vi "运维调试_养殖渭水采配水.vi"() -> ()   [LabVIEW 2016, in "PLC.lvlib"]
uses:
  PLC.lvlib
  control/switch.ctl
  <vilib>/Plasmionique/MB Master/MB_Master/MB_Master.lvclass
  <vilib>/Utility/miscctls.llb/LVPointTypeDef.ctl
  <vilib>/Plasmionique/MB Master/MB_Master_Serial/MB_Master_Serial.lvclass
  E:/Program Files (x86)/National Instruments/LabVIEW 2016/vi.lib/Plasmionique/MB Master/MB_Master/MB_Master.lvclass
  <vilib>/Plasmionique/MB Master/MB_Master_TCP/MB_Master_TCP.lvclass
  <vilib>/Plasmionique/MB Master/MB Master.lvlib
panel:
  out "告警":u16(ring) items=["无告警", "液位2异常告警", "进样失败告警", "阀1打开失败告警", "阀1关闭失败告警", "阀2打开失败告警", "阀2关闭失败告警"]
  in  "连接设置":bool
  out "水箱进样超时时间":i16
  out "水箱排液时间":i16
  out "水箱润洗超时时间":i16
  out "Registers":u16[](array[numeric])
  out "状态":u16(ring) items=["空闲", "忙碌"]
  in  "两通阀2":T1
  in  "两通阀1":T1
  out "采配水版本号":string
  out "配水时间":i16
  out "沉淀时间":i16 caption="多参测试、沉淀时间"
  out "管路润洗时间":i16
  out "多列列表框":i32(listbox)
  in  "隔膜泵":T1
  in  "返回":T1
  in  "参数设置":T1
  in  "启动":T1
  in  "停止":T1
  # "S"
  # "S"
  # "S"
  # "S"
  # "S"
  # "S"
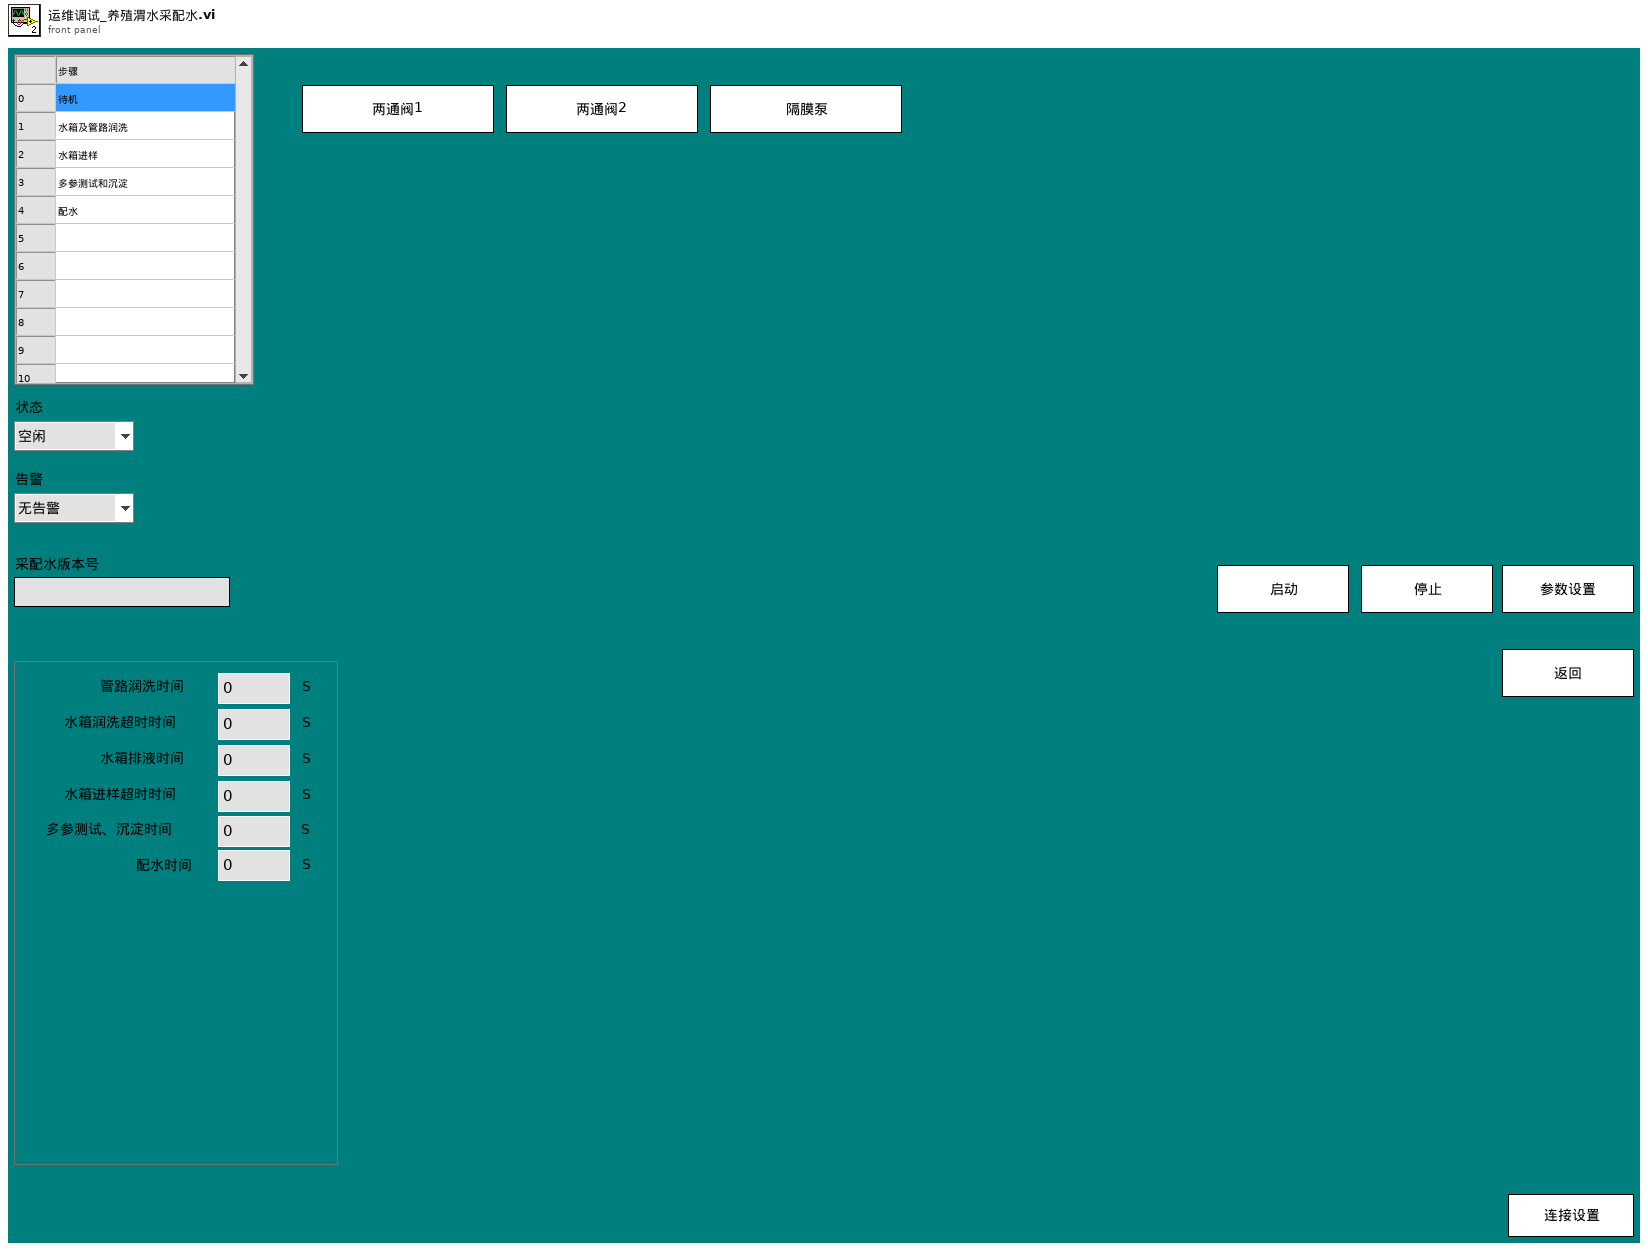
[diagram p1: front panel]
types:
  T1 = typedef "PLC.lvlib/switch.ctl" = bool
  T2 = typedef "参数.ctl" = cluster{"测试模式":enum16{"水样测试", "平行样测试", "集成干预测试", "加标回收"}, "参数启用":T3}
  T3 = typedef "启动参数.ctl" = cluster{"氨氮":bool, "总磷":bool, "总氮":bool, "多参数":bool, "CODmn":bool, "CODCr":bool, "氟化物":bool, "超标留样":bool, "重金属":bool, "挥发酚":bool}
  T4 = typedef "LVPointTypeDef.ctl" = cluster{"Horizontal":i16, "Vertical":i16}
  T5 = cluster{"R0":i16, "R1":i16, "R2":i16, "R3":i16, "R4":i16, "R5":i16, "R6":i16, "R7":i16, "R8":i16, "R9":i16, "R10":i16, "R11":i16, "R12":i16, "R13":i16, "R14":i16, "R15":i16, "R16":i16, "R17":i16, "R18":i16, "R19":i16, "R20":i16, "R21":i16, "R22":i16, "R23":i16, "R24":i16, "R25":i16, "R26":i16, "R27":i16, "R28":i16, "R29":i16, "R30":i16, "R31":i16, "R32":i16, "R33":i16, "R34":i16, "R35":i16, "R36":i16, "R37":i16, "R38":i16, "R39":i16, "R40":i16, "R41":i16, "R42":i16, "R43":i16, "R44":i16, "R45":i16, "R46":i16, "R47":i16, "R48":i16, "R49":i16, "R50":i16, "R51":i16, "R52":i16, "R53":i16, "R54":i16, "R55":i16, "R56":i16, "R57":i16, "R58":i16, "R59":i16, "R60":i16, "R61":i16, "R62":i16, "R63":i16, "R64":i16, "R65":i16, "R66":i16, "R67":i16, "R68":i16, "R69":i16, "R70":i16, "R71":i16, "R72":i16, "R73":i16, "R74":i16, "R75":i16, "R76":i16, "R77":i16, "R78":i16, "R79":i16}
  T6 = cluster{"seconds since 1Jan1904":timestamp, "table输入":string, string, "table输入":string}
  T7 = cluster{"命令":string, cluster{"starting address":u16, "holding register value":u16}}
  T8 = cluster{"命令":string, "数据":cluster{"starting address":u16, "holding register values":u16[]}}
  T9 = cluster{"测试模式":enum16{"水样测试", "平行样测试", "集成干预测试", "加标回收"}, "参数启用":T3}
  T10 = cluster{"baud rate (bps)":u32, "stop bits":u16, "parity":u16, "flow control":u16, "timeout":u32, "retries":i32}
  T11 = cluster{"starting address":u16, "holding register values":u16[]}
  T12 = cluster{"starting address":u16, "holding register value":u16}
  T13 = cluster{"starting address":u16, "coil values":bool[]}
  T14 = cluster{"连接类型":enum16{"串口", "TCP"}, "串口":string, "IP":string, "PORT":u16}
  T15 = cluster{"WORD[0]":u16, "WORD[1]":u16, "WORD[2]":u16, "WORD[3]":u16, "WORD[4]":u16, "WORD[5]":u16, "WORD[6]":u16, "WORD[7]":u16, "WORD[8]":u16, "WORD[9]":u16, "WORD[10]":u16, "WORD[11]":u16, "WORD[12]":u16, "WORD[13]":u16, "WORD[14]":u16, "WORD[15]":u16, "WORD[16]":u16, "WORD[17]":u16, "WORD[18]":u16, "WORD[19]":u16, "WORD[20]":u16, "WORD[21]":u16, "WORD[22]":u16, "WORD[23]":u16, "WORD[24]":u16, "WORD[25]":u16, "WORD[26]":u16, "WORD[27]":u16, "WORD[28]":u16, "WORD[29]":u16, "WORD[30]":u16, "WORD[31]":u16, "WORD[32]":u16, "WORD[33]":u16, "WORD[34]":u16, "WORD[35]":u16, "WORD[36]":u16, "WORD[37]":u16, "WORD[38]":u16, "WORD[39]":u16, "WORD[40]":u16, "WORD[41]":u16, "WORD[42]":u16, "WORD[43]":u16, "WORD[44]":u16, "WORD[45]":u16, "WORD[46]":u16, "WORD[47]":u16, "WORD[48]":u16, "WORD[49]":u16, "WORD[50]":u16, "WORD[51]":u16, "WORD[52]":u16, "WORD[53]":u16, "WORD[54]":u16, "WORD[55]":u16, "WORD[56]":u16, "WORD[57]":u16, "WORD[58]":u16, "WORD[59]":u16, "WORD[60]":u16, "WORD[61]":u16, "WORD[62]":u16, "WORD[63]":u16, "WORD[64]":u16, "WORD[65]":u16, "WORD[66]":u16, "WORD[67]":u16, "WORD[68]":u16, "WORD[69]":u16, "WORD[70]":u16, "WORD[71]":u16, "WORD[72]":u16, "WORD[73]":u16, "WORD[74]":u16, "WORD[75]":u16, "WORD[76]":u16, "WORD[77]":u16, "WORD[78]":u16, "WORD[79]":u16}
  T16 = cluster{"Registers[0]":u16, "Registers[1]":u16, "Registers[2]":u16, "Registers[3]":u16, "Registers[4]":u16, "Registers[5]":u16, "Registers[6]":u16, "Registers[7]":u16, "Registers[8]":u16, "Registers[9]":u16, "Registers[10]":u16, "Registers[11]":u16, "Registers[12]":u16, "Registers[13]":u16, "Registers[14]":u16, "Registers[15]":u16, "Registers[16]":u16, "Registers[17]":u16, "Registers[18]":u16, "Registers[19]":u16, "Registers[20]":u16, "Registers[21]":u16, "Registers[22]":u16, "Registers[23]":u16, "Registers[24]":u16, "Registers[25]":u16, "Registers[26]":u16, "Registers[27]":u16, "Registers[28]":u16, "Registers[29]":u16, "Registers[30]":u16, "Registers[31]":u16, "Registers[32]":u16, "Registers[33]":u16, "Registers[34]":u16, "Registers[35]":u16, "Registers[36]":u16}
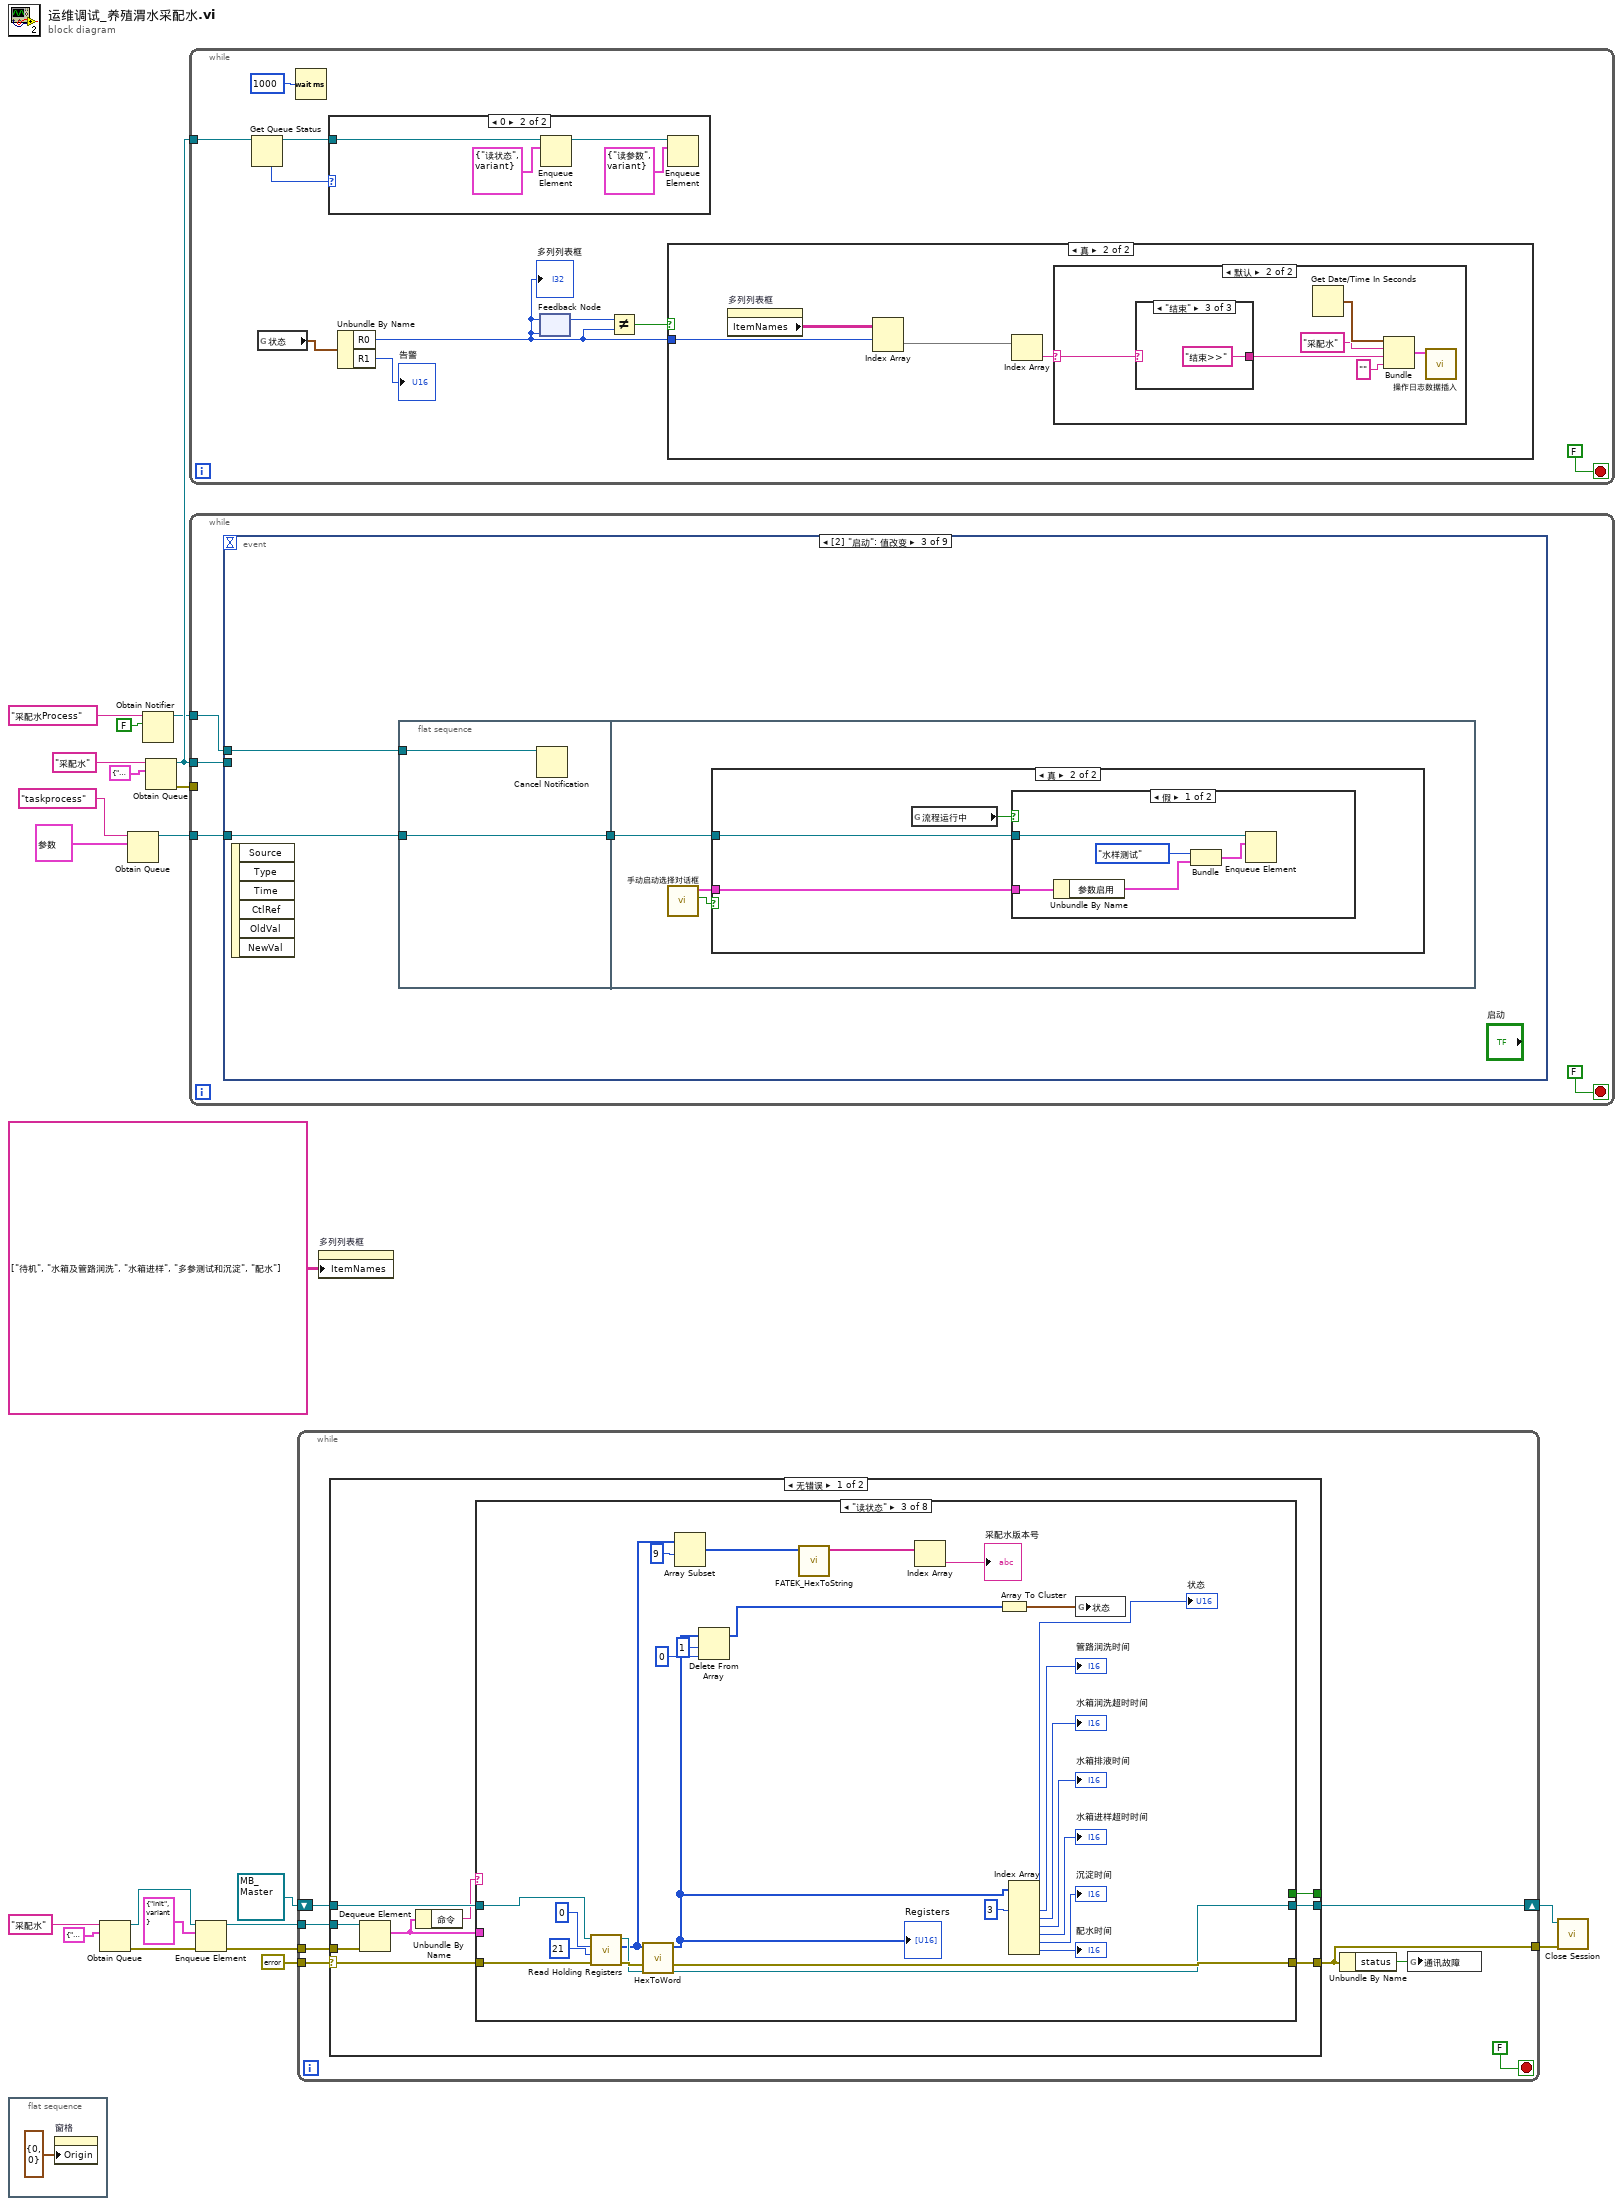
[diagram p0: block diagram]
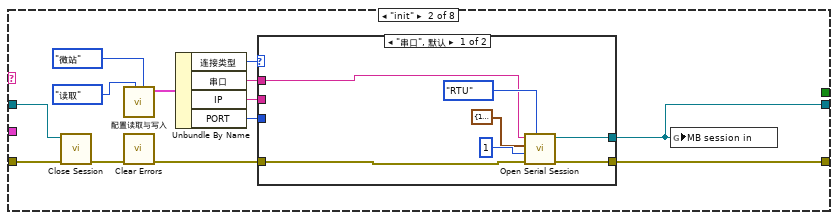
[diagram p3: hidden frame]
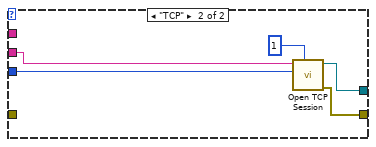
[diagram p4: hidden frame]
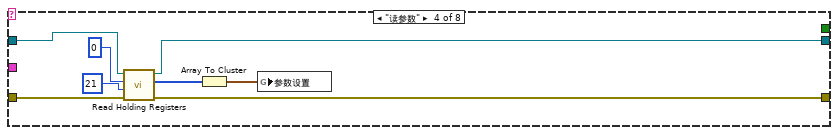
[diagram p5: hidden frame]
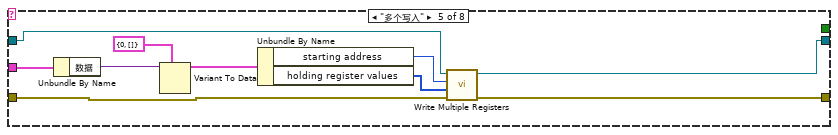
[diagram p6: hidden frame]
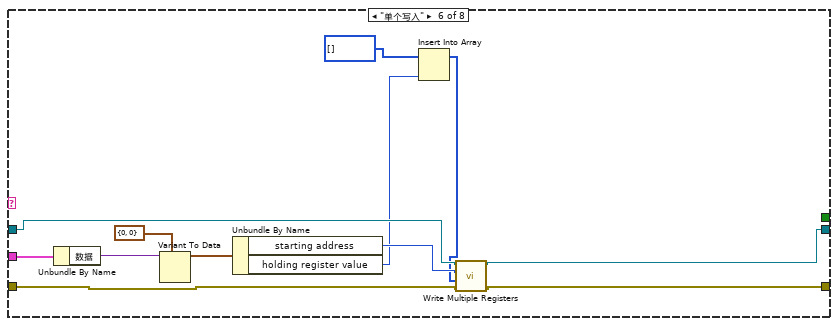
[diagram p7: hidden frame]
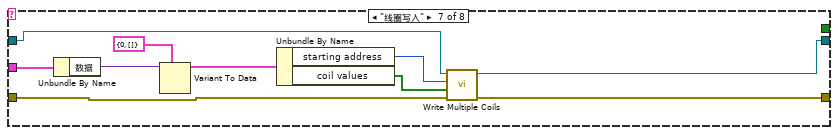
[diagram p8: hidden frame]
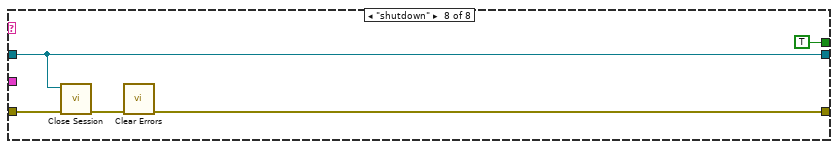
[diagram p9: hidden frame]
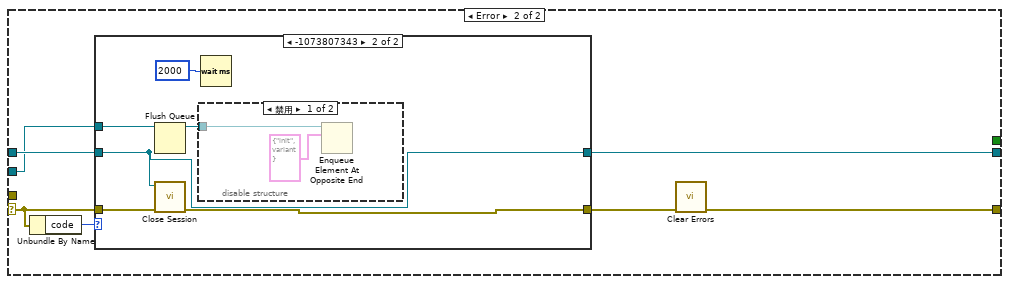
[diagram p10: hidden frame]
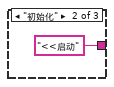
[diagram p17: hidden frame]
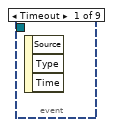
[diagram p18: hidden frame]
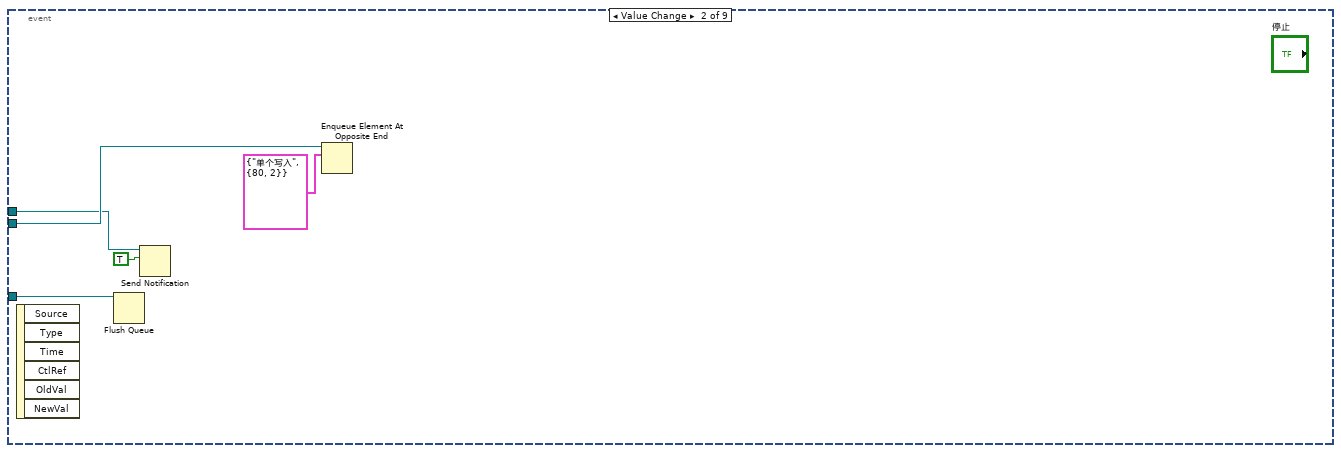
[diagram p19: hidden frame]
diagram:
  n1 = flat-sequence {
    frame #0 {
      n2 = property on="窗格" class="Pane"("Origin"=T4 {"Horizontal"=0, "Vertical"=0} ("原点")) -> ()  [unwired: 2 in, 2 out]
    }
  }
  n3 = Obtain Queue(name (unnamed)="采配水" ("名称（未命名）"), element data type=cluster{"命令":string, "数据":variant} {"命令"="", "数据"=variant}) -> (queue out=w12:refnum<queue>, error out=w11:errorcluster)  [unwired: 3 in, 1 out]
  n4 = Obtain Queue(name (unnamed)="taskprocess" ("名称（未命名）"), element data type=T2 {"测试模式"=enum."水样测试", "参数启用"={"氨氮"=FALSE, "总磷"=FALSE, "总氮"=FALSE, "多参数"=FALSE, "CODmn"=FALSE, "CODCr"=FALSE, "氟化物"=FALSE, "超标留样"=FALSE, "重金属"=FALSE, "挥发酚"=FALSE}} ("参数")) -> (queue out=w2:refnum<queue>)  [unwired: 3 in, 2 out]
  n5 = Obtain Notifier(name (unnamed)="采配水Process" ("名称（未命名）"), notification data type=FALSE) -> (notifier out=w15:refnum<notifier>)  [unwired: 2 in, 2 out]
  n6 = Obtain Queue(name (unnamed)="采配水" ("名称（未命名）"), element data type=cluster{"命令":string, "数据":variant} {"命令"="", "数据"=variant}) -> (queue out=w19:refnum<queue>, error out=w20:errorcluster)  [unwired: 3 in, 1 out]
  n7 = while {
    tunnel: w19 -> [w32]
    stop <- FALSE stop-if-true
    n8 = Get Queue Status(queue=w32) -> (queue out=w27:refnum<queue>, # elements in queue=w26:i32)  [unwired: 2 in, 6 out]
    n9 = global read "采配水全局变量.vi" "状态"() -> (w31:T5)
    n10 = Wait (ms)(milliseconds to wait=u32 1000 ("等待时间（毫秒）")) -> ()  [unwired: 1 out]
    n11 = case shown="0" w26 {
      tunnel: w27 -> [_ w37]
      frame Default {
      }
      frame 0 {
        n12 = Enqueue Element(queue=w37, element=cluster{"命令":string, "数据":variant} {"命令"="读状态", "数据"=variant} ("元素")) -> (queue out=w34:refnum<queue>)  [unwired: 2 in, 2 out]
        n13 = Enqueue Element(queue=w34, element=cluster{"命令":string, "数据":variant} {"命令"="读参数", "数据"=variant} ("元素")) -> ()  [unwired: 2 in, 3 out]
      }
    }
    n14 = Unbundle By Name(w31) -> ("R0"=w25:i16, "R1"=→"告警":i16)
    "多列列表框" <- w25
    n15 = feedback-in #1(w25) -> ()
    n16 = feedback #1(w25) -> (w28:i16)
    n17 = Not Equal?(x=w28, y=w25) -> (x != y?=w30:bool)
    n18 = case shown="真" w30 {
      tunnel: w25 -> [_ w40]
      frame False {
      }
      frame True {
        n19 = property on="多列列表框" class="MCListbox (严格)"() -> ("ItemNames"=w41:string[][])  [unwired: 2 in, 2 out]
        n20 = Index Array(array=w41, index (row)=w40) -> (element=w39:string[])  [unwired: 1 in]
        n21 = Index Array(array=w39) -> (element=w38:string)  [unwired: 1 in]
        n22 = case shown="默认" w38 {
          selector: w38 -> [_ w44]
          frame "待机" {
          }
          frame Default {
            n23 = case shown="\"结束\"" w44 {
              selector: w44 -> [w48 _ _]
              tunnel: [w48 "<<启动" "结束>>"] -> w43
              frame Default {
              }
              frame "初始化" {
              }
              frame "结束" {
              }
            }
            n24 = Get Date/Time In Seconds() -> (seconds since 1Jan1904=w47:timestamp)
            n25 = Bundle("seconds since 1Jan1904"=w47, "table输入"="采配水", w43, "table输入"="") -> (w42:T6)  [unwired: 1 in]
            n26 = call "操作日志数据插入.vi"("data"=w42) -> ()  [unwired: 9 in, 1 out]
          }
        }
      }
    }
  }
  n27 = while {
    tunnel: w19 -> [w53]
    tunnel: w20 -> [_]
    tunnel: w15 -> [w52]
    tunnel: w2 -> [w51]
    stop <- FALSE stop-if-true
    n28 = event shown="[2] \"启动\": 值改变" {
      selector: _ -> [_ _ _ _ _ _ _ _ _]
      dyn-events: _ -> [_ _ _ _ _ _ _ _ _]
      timeout: _ -> [_ _ _ _ _ _ _ _ _]
      tunnel: w53 -> [_ w58 _ w85 w98 _ _ _ w110]
      tunnel: w52 -> [_ w57 w62 _ _ _ _ _ _]
      tunnel: w51 -> [_ w55 w60 _ _ _ _ _ _]
      event Timeout {
        n29 = event-data() -> ()  [unwired: 1 in, 3 out]
      }
      event Value Change {
        n30 = event-data() -> ()  [unwired: 1 in, 6 out]
        n31 = Flush Queue(queue=w55) -> ()  [unwired: 1 in, 3 out]
        n32 = Send Notification(notification=TRUE ("通知"), notifier=w57) -> ()  [unwired: 1 in, 2 out]
        n33 = Enqueue Element At Opposite End(queue=w58, element=T7 {"命令"="单个写入", {"starting address"=80, "holding register value"=2}} ("元素")) -> ()  [unwired: 2 in, 3 out]
      }
      event Value Change {
        n34 = event-data() -> ()  [unwired: 1 in, 6 out]
        n35 = flat-sequence {
          tunnel: w62 -> [w64]
          tunnel: [w63] -> w61
          tunnel: w60 -> [w63]
          tunnel: w61 -> [w65]
          frame #0 {
            n36 = Cancel Notification(0:w64) -> ()  [unwired: 1 in, 3 out]
          }
          frame #1 {
            n37 = call "手动启动选择对话框.vi"() -> ("确定"=w67:bool, "输出簇"=w66:cluster{"参数启用":T3})  [unwired: 10 in]
            n38 = case shown="真" w67 {
              tunnel: w66 -> [_ w70]
              tunnel: w65 -> [_ w69]
              frame False {
              }
              frame True {
                n39 = global read "采配水全局变量.vi" "流程运行中"() -> (w68:bool)
                n40 = case shown="假" w68 {
                  tunnel: w70 -> [w73 _]
                  tunnel: w69 -> [w75 _]
                  frame False {
                    n41 = Unbundle By Name(w73) -> ("参数启用"=w72:T3)
                    n42 = Bundle("测试模式"=enum16{"水样测试", "平行样测试", "集成干预测试", "加标回收"}."水样测试", "参数启用"=w72) -> (w71:T9)  [unwired: 1 in]
                    n43 = Enqueue Element(queue=w75, element=w71) -> ()  [unwired: 2 in, 3 out]
                  }
                  frame True {
                    n44 = One Button Dialog(message="流程已启动，无需重复启动！" ("消息")) -> ()  [unwired: 1 in, 1 out]
                  }
                }
              }
            }
          }
        }
      }
      event "管路润洗时间", "沉淀时间", "配水时间", "水箱润洗超时时间", "水箱排液时间", "水箱进样超时时间": Value Change {
        n45 = event-data() -> ("CtlRef"=w81:refnum<vi>)  [unwired: 1 in, 5 out]
        n46 = property class="DigNum (严格)"(reference=w81) -> ("Label.Text"=w80:string)  [unwired: 1 in, 2 out]
        n47 = case shown="\"配水时间\"" w80 {
          tunnel: [u16 3 ("数据.starting address") u16 4 ("数据.starting address") u16 5 ("数据.starting address") u16 6 ("数据.starting address") u16 7 ("数据.starting address") u16 8 ("数据.starting address")] -> w78
          tunnel: [w86 w89 w91 w92 w94 w97] -> w79
          frame "管路润洗时间", Default {
            n48 = local read "管路润洗时间"() -> (w86:i16)
          }
          frame "水箱润洗超时时间" {
            n49 = local read "水箱润洗超时时间"() -> (w89:i16)
          }
          frame "水箱排液时间" {
            n50 = local read "水箱排液时间"() -> (w91:i16)
          }
          frame "水箱进样超时时间" {
            n51 = local read "水箱进样超时时间"() -> (w92:i16)
          }
          frame "沉淀时间" {
            n52 = local read "沉淀时间"() -> (w94:i16)
          }
          frame "配水时间" {
            n53 = local read "配水时间"() -> (w97:i16)
          }
        }
        n54 = Build Array(w79) -> (w77:i16[])
        n55 = call "WordToHex.vi"("WORD"=w77) -> ("数组"=w82:u16[])  [unwired: 10 in]
        n56 = Bundle By Name(cluster=T8 {"命令"="多个写入", "数据"={"starting address"=0, "holding register values"=[]}} ("元素"), "数据.starting address"=w78, "数据.holding register values"=w82) -> (w83:T8)
        n57 = Enqueue Element At Opposite End(queue=w85, element=w83) -> ()  [unwired: 2 in, 3 out]
      }
      event "连接设置": Value Change {
        n58 = event-data() -> ()  [unwired: 1 in, 6 out]
        n59 = call "连接配置对话框.vi"("类别"=enum16{"微站", "固定站"}."微站") -> ("check？"=w100:bool)  [unwired: 18 in]
        n60 = case shown="真" w100 {
          tunnel: w98 -> [_ w102]
          frame False {
          }
          frame True {
            n61 = Enqueue Element(queue=w102, element=cluster{"命令":string, "数据":variant} {"命令"="init", "数据"=variant} ("元素")) -> ()  [unwired: 2 in, 3 out]
          }
        }
      }
      event "管路润洗时间", "沉淀时间", "配水时间", "水箱润洗超时时间", "水箱排液时间", "水箱进样超时时间": Mouse Down {
        n62 = event-data() -> ("CtlRef"=w106:refnum<vi>)  [unwired: 1 in, 7 out]
        n63 = property class="DigNum (严格)"(reference=w106) -> (reference out=w104:refnum<vi>, "Value"=w105:i16)  [unwired: 1 in, 1 out]
        n64 = call "数字键盘.vi"("OldNumber"=w105) -> ("NewNumber"=w103:sgl)
        n65 = property class="DigNum (严格)"(reference=w104, "Val(Sgnl)"=w103) -> ()  [unwired: 1 in, 2 out]
      }
      event Value Change {
        n66 = event-data() -> ()  [unwired: 1 in, 6 out]
        n67 = property on="窗格" class="Pane"("Origin"=T4 {"Horizontal"=0, "Vertical"=628} ("原点")) -> ()  [unwired: 2 in, 2 out]
      }
      event Value Change {
        n68 = event-data() -> ()  [unwired: 1 in, 6 out]
        n69 = property on="窗格" class="Pane"("Origin"=T4 {"Horizontal"=0, "Vertical"=0} ("原点")) -> ()  [unwired: 2 in, 2 out]
      }
      event Value Change {
        n70 = event-data() -> ("CtlRef"=w115:refnum<vi>, "NewVal"=w113:T1)  [unwired: 1 in, 4 out]
        n71 = property class="Bool (严格)"(reference=w115) -> ("Label.Text"=w114:string)  [unwired: 1 in, 2 out]
        n72 = case shown="\"两通阀1\", 默认" w114 {
          tunnel: w113 -> [w119 w123 w127]
          tunnel: [w118 w122 w126] -> w112
          frame "两通阀1", Default {
            n73 = Select(t=u16 3 ("starting address"), s=w119, f=u16 4 ("starting address")) -> (s? t:f=w118:u16)
          }
          frame "两通阀2" {
            n74 = Select(t=u16 5 ("starting address"), s=w123, f=u16 6 ("starting address")) -> (s? t:f=w122:u16)
          }
          frame "隔膜泵" {
            n75 = Select(t=u16 7 ("starting address"), s=w127, f=u16 8 ("starting address")) -> (s? t:f=w126:u16)
          }
        }
        n76 = Build Array(w112) -> (w111:u16[])
        n77 = Bundle By Name(cluster=T8 {"命令"="多个写入", "数据"={"starting address"=0, "holding register values"=[]}} ("元素"), "数据.starting address"=u16 80, "数据.holding register values"=w111) -> (w109:T8)
        n78 = Enqueue Element(queue=w110, element=w109) -> ()  [unwired: 2 in, 3 out]
      }
    }
  }
  n79 = Enqueue Element(queue=w12, element=cluster{"命令":string, "数据":variant} {"命令"="init", "数据"=variant} ("元素"), error in (no error)=w11) -> (queue out=w7:refnum<queue>, error out=w9:errorcluster)  [unwired: 1 in, 1 out]
  n80 = while {
    tunnel: w7 -> [w134]
    tunnel: w9 -> [w133]
    shift-right: [w137] -> w4
    shift-left: refnum<class "MB_Master.lvclass"> refnum ("MB session in") -> [w136]
    tunnel: errorcluster {"status"=FALSE, "code"=0, "source"=""} ("error out") -> [w135]
    tunnel: [w132] -> w5
    stop <- FALSE stop-if-true
    n81 = case shown="无错误" w135 {
      selector: w135 -> [w143 w247]
      tunnel: [w146 w246] -> w137
      tunnel: w136 -> [w145 w248]
      tunnel: [w144 w244] -> w132
      tunnel: w134 -> [w140 w243]
      tunnel: w133 -> [w139 _]
      tunnel: [w141 _] -> _
      frame No Error {
        n82 = Dequeue Element(queue=w140, error in (no error)=w139) -> (element=w138:cluster{"命令":string, "数据":variant})  [unwired: 1 in, 3 out]
        n83 = Unbundle By Name(w138) -> ("命令"=w142:string)
        n84 = case shown="\"读状态\"" w142 {
          tunnel: [w148 w151 w180 w200 w212 w222 w234 w239] -> w146
          tunnel: w145 -> [w148 w159 w194 w205 w215 w223 w237 w239]
          tunnel: [w147 w150 w181 w199 w213 w221 w235 w238] -> w144
          tunnel: w143 -> [w147 w161 w197 w204 w214 w220 w236 w240]
          tunnel: [_ _ _ _ _ _ _ TRUE] -> w141
          tunnel: w138 -> [_ _ _ _ w211 w227 w233 _]
          frame "idle", Default {
          }
          frame "init" {
            n85 = call-dynamic "Close Session.vi"("error in (no error)"=w161, "MB session in"=w159) -> ("error out"=w160:errorcluster)  [unwired: 9 in]
            n86 = call "配置读取与写入.vi"("类别"=enum16{"微站", "固定站"}."微站", "功能"=enum16{"读取", "写入"}."读取") -> ("连接配置 2"=w157:T14)  [unwired: 8 in, 1 out]
            n87 = call <vilib>:"Clear Errors.vi"("error in (no error)"=w160) -> ("error out"=w149:errorcluster)  [unwired: 5 in, 1 out]
            n88 = Unbundle By Name(w157) -> ("连接类型"=w154:enum16{"串口", "TCP"}, "串口"=w156:string, "IP"=w153:string, "PORT"=w152:u16)
            n89 = case shown="\"串口\", 默认" w154 {
              tunnel: [w168 w170] -> w150
              tunnel: w149 -> [w162 _]
              tunnel: [w164 w171] -> w151
              tunnel: w156 -> [w163 _]
              tunnel: w153 -> [_ w173]
              tunnel: w152 -> [_ w172]
              frame "串口", Default {
                n90 = call <vilib>:"Open Serial Session.vi"("Mode (RTU)"=enum16{"RTU", "ASCII"}."RTU", "Error in"=w162, "Slave ID"=u8 1, "Serial Config"=T10 {"baud rate (bps)"=115200, "stop bits"=10, "parity"=0, "flow control"=0, "timeout"=500, "retries"=1}, "VISA Resource"=w163) -> ("Error out"=w168:errorcluster, "MB_Serial session"=w164:refnum<class "MB_Master_Serial.lvclass">)  [unwired: 5 in]
              }
              frame "TCP" {
                n91 = call <vilib>:"Open TCP Session.vi"("Slave ID (255)"=u8 1, "Port (502)"=w172, "IP Address"=w173) -> ("error out"=w170:errorcluster, "MB_TCP session"=w171:refnum<class "MB_Master_TCP.lvclass">)  [unwired: 7 in]
              }
            }
            n92 = global write "采配水全局变量.vi" "MB session in"(w151) -> ()
          }
          frame "读状态" {
            n93 = call <vilib>:"Read Holding Registers.vi"("error in (no error)"=w197, "quantity"=u16 21 ("number of holding registers"), "starting address"=u16 0, "MB session in"=w194) -> ("error out"=w181:errorcluster, "Registers"=w179:u16[], "MB session out"=w180:refnum<class "MB_Master.lvclass">)  [unwired: 5 in]
            n94 = call "HexToWord.vi"("数组"=w179) -> ("WORD"=w178:u16[])  [unwired: 10 in]
            "Registers" <- w178
            n95 = Array Subset(array=w179, index=9 ("索引")) -> (w192:u16[])  [unwired: 1 in]
            n96 = Delete From Array(array=w178, length=1 ("长度"), index=0 ("索引")) -> (array with subset deleted=w175:u16[])  [unwired: 1 out]
            n97 = call "FATEK_HexToString.vi"("数组"=w192) -> ("STRING"=w191:string[])  [unwired: 10 in]
            n98 = Index Array(array=w191) -> (element=→"采配水版本号":string)  [unwired: 1 in]
            n99 = Array To Cluster(array=w175) -> (cluster=w188:T15)
            n100 = Index Array(array=w178, index #2=3 ("索引")) -> (element #1=→"状态":u16, element #2=→"管路润洗时间":u16, element #3=→"水箱润洗超时时间":u16, element #4=→"水箱排液时间":u16, element #5=→"水箱进样超时时间":u16, element #6=→"沉淀时间":u16, element #7=→"配水时间":u16)  [unwired: 6 in]
            n101 = global write "采配水全局变量.vi" "状态"(w188) -> ()
          }
          frame "读参数" {
            n102 = call <vilib>:"Read Holding Registers.vi"("error in (no error)"=w204, "quantity"=u16 21 ("number of holding registers"), "starting address"=u16 0, "MB session in"=w205) -> ("error out"=w199:errorcluster, "Registers"=w201:u16[], "MB session out"=w200:refnum<class "MB_Master.lvclass">)  [unwired: 5 in]
            n103 = Array To Cluster(array=w201) -> (cluster=w198:T16)
            n104 = global write "采配水全局变量.vi" "参数设置"(w198) -> ()
          }
          frame "多个写入" {
            n105 = Unbundle By Name(w211) -> ("数据"=w210:variant)
            n106 = Variant To Data(type=T11 {"starting address"=0, "holding register values"=[]}, Variant=w210) -> (data=w208:T11)  [unwired: 1 in, 1 out]
            n107 = Unbundle By Name(w208) -> ("starting address"=w207:u16, "holding register values"=w206:u16[])
            n108 = call <vilib>:"Write Multiple Registers.vi"("error in (no error)"=w214, "values"=w206, "starting address"=w207, "MB session in"=w215) -> ("error out"=w213:errorcluster, "MB session out"=w212:refnum<class "MB_Master.lvclass">)  [unwired: 6 in]
          }
          frame "单个写入" {
            n109 = Unbundle By Name(w227) -> ("数据"=w226:variant)
            n110 = Variant To Data(type=T12 {"starting address"=0, "holding register value"=0}, Variant=w226) -> (data=w224:T12)  [unwired: 1 in, 1 out]
            n111 = Unbundle By Name(w224) -> ("starting address"=w219:u16, "holding register value"=w217:u16)
            n112 = Insert Into Array(array=u16[] [] ("holding register values"), new element=w217) -> (w216:u16[])  [unwired: 1 in]
            n113 = call <vilib>:"Write Multiple Registers.vi"("error in (no error)"=w220, "values"=w216, "starting address"=w219, "MB session in"=w223) -> ("error out"=w221:errorcluster, "MB session out"=w222:refnum<class "MB_Master.lvclass">)  [unwired: 6 in]
          }
          frame "线圈写入" {
            n114 = Unbundle By Name(w233) -> ("数据"=w232:variant)
            n115 = Variant To Data(type=T13 {"starting address"=0, "coil values"=[]}, Variant=w232) -> (data=w230:T13)  [unwired: 1 in, 1 out]
            n116 = Unbundle By Name(w230) -> ("starting address"=w229:u16, "coil values"=w228:bool[])
            n117 = call <vilib>:"Write Multiple Coils.vi"("error in (no error)"=w236, "values"=w228, "starting address"=w229, "MB session in"=w237) -> ("error out"=w235:errorcluster, "MB session out"=w234:refnum<class "MB_Master.lvclass">)  [unwired: 6 in]
          }
          frame "shutdown" {
            n118 = call-dynamic "Close Session.vi"("error in (no error)"=w240, "MB session in"=w239) -> ("error out"=w241:errorcluster)  [unwired: 9 in]
            n119 = call <vilib>:"Clear Errors.vi"("error in (no error)"=w241) -> ("error out"=w238:errorcluster)  [unwired: 5 in, 1 out]
          }
        }
      }
      frame Error {
        n120 = Unbundle By Name(w247) -> ("code"=w249:i32)
        n121 = case shown="-1073807343" w249 {
          tunnel: w248 -> [w251 w255]
          tunnel: w247 -> [w250 w257]
          tunnel: [w250 w256] -> w245
          tunnel: [w251 w255] -> w246
          tunnel: w243 -> [_ w254]
          frame Default {
          }
          frame -1073807343 {
            n122 = Flush Queue(queue=w254) -> (queue out=w253:refnum<queue>)  [unwired: 1 in, 2 out]
            n123 = call-dynamic "Close Session.vi"("error in (no error)"=w257, "MB session in"=w255) -> ("error out"=w256:errorcluster)  [unwired: 9 in]
            n124 = disable-structure shown="禁用" {
              disable-tunnel: w253 -> [w258 _]
              frame Disabled {
                n125 = Enqueue Element At Opposite End(queue=w258, element=cluster{"命令":string, "数据":variant} {"命令"="init", "数据"=variant} ("元素")) -> ()  [unwired: 2 in, 3 out]
              }
              frame Enabled {
              }
            }
            n126 = Wait (ms)(milliseconds to wait=u32 2000 ("等待时间（毫秒）")) -> ()  [unwired: 1 out]
          }
        }
        n127 = call <vilib>:"Clear Errors.vi"("error in (no error)"=w245) -> ("error out"=w244:errorcluster)  [unwired: 5 in, 1 out]
      }
    }
    n128 = Unbundle By Name(w132) -> ("status"=w130:bool)
    n129 = global write "采配水全局变量.vi" "通讯故障"(w130) -> ()
  }
  n130 = property on="多列列表框" class="MCListbox (严格)"("ItemNames"=string[][] [["待机"], ["水箱及管路润洗"], ["水箱进样"], ["多参测试和沉淀"], ["配水"]] ("项名")) -> ()  [unwired: 2 in, 2 out]
  n131 = call-dynamic "Close Session.vi"("error in (no error)"=w5, "MB session in"=w4) -> ()  [unwired: 9 in, 1 out]
